vi "Write tSignalonTreeElements_Core.vi"(8 "error in (no error)":errorcluster, 9 "System_settings IN":T1={"Units in the system"=[], "dBase names by units"=[], "TCP/IP processing units addresses"=[], "TCP/IP server address"="", "dBase User Name_Cli"="codis_cli", "dBase User Password_Cli"="codis_cli", "dBase User Name_Med"="codis_med_wrt", "dBase User Password_Med"="codis_med_wrt", "Sampling rate [Hz]"=0.0, "FTP Server User name, cRIO"="", "FTP Server Password, cRIO"="", "OnScreenKeyboardPopUp"=FALSE, "Number of points to collect"=0, "Main Window has title bar?"=FALSE, "Demo?"=FALSE, "dBase - Limit # of  elements to read"=0, "dBase Backup"={"dBase Backup Base Folder"="c:\\codis\\backup\\", "Remote dBase Backup Configured?"=TRUE}, "System Status"={"System Monitor Refresh Rate (ms)"=10000, "System Status Log  File"="c:\\codis\\system_info.txt", "Max number of elements to read\n"=26611200}, "Number of points to average for stationary state"=[60], "Number of points to collect for saving waveforms per channel"=[60], "Sources per Unit"=[], "TCP/IP_client_mediator_communication ports"=2058, "TCP/IP processing_units _mediator_communication ports"=2055}, 10 "1D array of Pan Cluster IN":T4[](array[typedef]) {"Absolute Minimum Air Gap per Plane"."Absolute AG Minimum Pole Number" format="%.3f"; "Absolute Minimum Air Gap per Plane"."Absolute AG Minimum Value" format="%.3f"; "Magnetic Field Data"."Maximum by Pole Number" format="%.3f"; "Air Gap Data"."Minimum by Pole Number" format="%.3f"; "Orbit(s) - XY"."Orbit XY Graphs (Synthesized from Selected Harmonics and DC)"."?" format="%.3f"; "Orbit(s) - XY"."Orbit XY Graphs (Synthesized from Selected Harmonics and DC)"."?" format="%.3f"; "Orbit(s) - XY"."Orbit XY Graphs (Glided and Averaged on One Revolution)"."?" format="%.3f"; "Orbit(s) - XY"."Orbit XY Graphs (Glided and Averaged on One Revolution)"."?" format="%.3f"; "Orbit(s) - XY"."Orbit XY Graphs (Unaveraged)"."?" format="%.3f"; "Orbit(s) - XY"."Orbit XY Graphs (Unaveraged)"."?" format="%.3f"}) -> ()   [LabVIEW 2014]
uses:
  common/typedefs/Pan_Cluster_Core.ctl
  common/typedefs/Condition_Vector_Cluster_Core.ctl
  common/typedefs/Unit_Names_Core.ctl
  common/typedefs/Data_Sources_Core.ctl
  common/typedefs/System_Settings_Cluster_Client_Mediator_Core.ctl
  <vilib>/addons/database/Connection.llb/DB Tools Open Connec (String).vi
  <vilib>/addons/database/_DB Variant To Data/Database Variant To Data.xnode
  <vilib>/addons/database/NI_Database_API.lvlib
panel:
  out "SignalLabel OUT":string[](array[string])
  out "TreeCategoryName":string[](array[string])
  out "idtTreeCategories OUT":u32[](array[numeric])
  out "TreeCategoryLabel":string[](array[string])
  out "error out 2":errorcluster
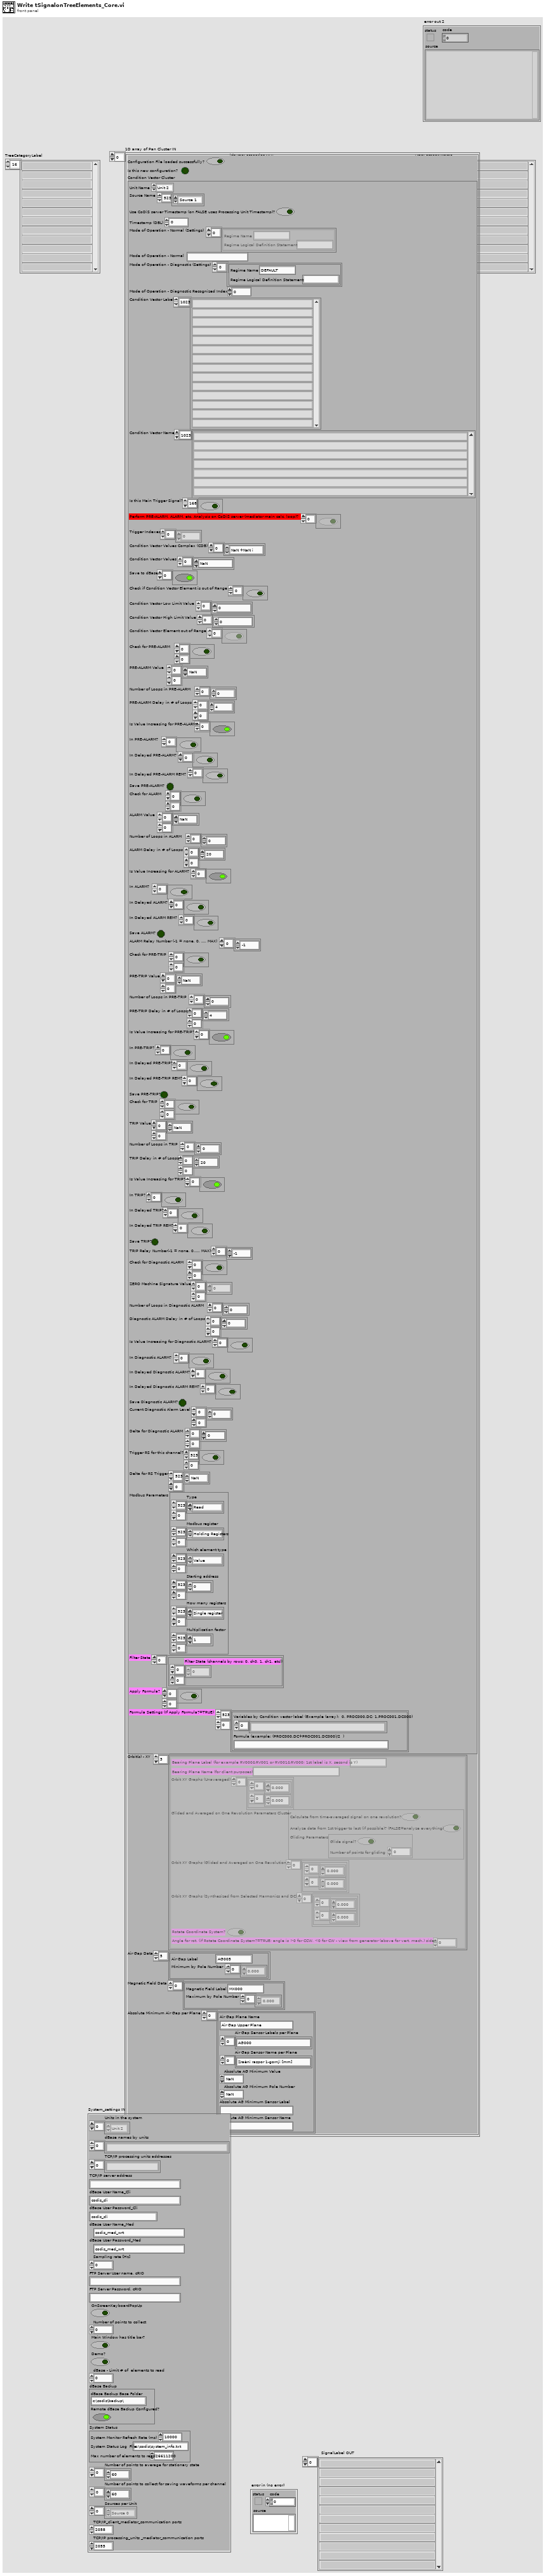
[diagram p1: front panel]
types:
  T1 = typedef "System_Settings_Cluster_Client_Mediator_Core.ctl" = cluster{"Units in the system":T2[], "dBase names by units":string[], "TCP/IP processing units addresses":string[], "TCP/IP server address":string, "dBase User Name_Cli":string, "dBase User Password_Cli":string, "dBase User Name_Med":string, "dBase User Password_Med":string, "Sampling rate [Hz]":dbl, "FTP Server User name, cRIO":string, "FTP Server Password, cRIO":string, "OnScreenKeyboardPopUp":bool, "Number of points to collect":u32, "Main Window has title bar?":bool, "Demo?":bool, "dBase - Limit # of  elements to read":u32, "dBase Backup":cluster{"dBase Backup Base Folder":string, "Remote dBase Backup Configured?":bool}, "System Status":cluster{"System Monitor Refresh Rate (ms)":u32, "System Status Log  File":string, "Max number of elements to read\n":i64}, "Number of points to average for stationary state":i32[], "Number of points to collect for saving waveforms per channel":i32[], "Sources per Unit":T3[], "TCP/IP_client_mediator_communication ports":u16, "TCP/IP processing_units _mediator_communication ports":u16}
  T2 = typedef "Unit_Names_Core.ctl" = enum16{"Not used", "Unit 1", "Unit 2", "Unit 3", "Unit 4", "Unit 5", "Unit 6", "Unit 7", "Unit 8", "Unit 9"}
  T3 = typedef "Data_Sources_Core.ctl" = enum16{"Not Used", "Source 0", "Source 1", "Source 2", "Source 3", "Source 4", "Source 5", "Source 6", "Source 7", "Source 8", "Source 9", "Source 10", "Source 11", "Source 12", "Source 13", "Source 14", "Source 15", "Source 16", "Source 17", "Source 18", "Source 19", "Source 20"}
  T4 = typedef "Pan_Cluster_Core.ctl" = cluster{"Configuration File loaded successfully?":bool, "Is this new configuration?":bool, "Condition Vector Cluster":T5, "Orbit(s) - XY":cluster{"Bearing Plane Label (for example RV000&RV001 or RV001&RV000; 1st label is X, second is Y)":string, "Bearing Plane Name (for client purposes)":string, "Orbit XY Graphs (Unaveraged)":cluster{sgl[], sgl[]}[], "Glided and Averaged on One Revolution Parameters Cluster":cluster{"Calculate from time-averaged signal on one revolution?":bool, "Analyze data from 1st trigger to last (if possible)? (FALSE=analyze everything)":bool, "Gliding Parameters":cluster{"Glide signal?":bool, "Number of points for gliding":u16}}, "Orbit XY Graphs (Glided and Averaged on One Revolution)":cluster{sgl[], sgl[]}[], "Orbit XY Graphs (Synthesized from Selected Harmonics and DC)":cluster{sgl[], sgl[]}[], "Rotate Coordinate System?":bool, "Angle for rot. (if Rotate Coordinate System?=TRUE; angle is >0 for CCW, <0 for CW - view from generator (above for vert. mach.) side)":sgl}[], "Air Gap Data":cluster{"Air Gap Label":string, "Minimum by Pole Number":sgl[]}[], "Magnetic Field Data":cluster{"Magnetic Field Label":string, "Maximum by Pole Number":sgl[]}[], "Absolute Minimum Air Gap per Plane":cluster{"Air Gap Plane Name":string, "Air Gap Sensor Labels per Plane":string[], "Air Gap Sensor Name per Plane":string[], "Absolute AG Minimum Value":sgl, "Absolute AG Minimum Pole Number":sgl, "Absolute AG Minimum Sensor Label":string, "Absolute AG Minimum Sensor Name":string}[]}
  T5 = typedef "Condition_Vector_Cluster_Core.ctl" = cluster{"Unit Name":T2, "Source Name":T3[], "Use CoDiS server Timestamp (on FALSE uses Processing Unit Timestamp)?":bool, "Timestamp (DBL)":dbl, "Mode of Operation - Normal (Settings)":cluster{"Regime Name":string, "Regime Logical Definition Statement":string}[], "Mode of Operation - Normal":string, "Mode of Operation - Diagnostic (Settings)":cluster{"Regime Name":string, "Regime Logical Definition Statement":string}[], "Mode of Operation - Diagnostic Recognized Index":i16, "Condition Vector Label":string[], "Condition Vector Name":string[], "Is this Main Trigger Signal?":bool[], "Perform PRE-ALARM, ALARM, etc. Analysis on CoDiS server (mediator main calc. loop)?":bool[], "Trigger Indexes":u32[], "Condition Vector Values Complex (CDB)":cdb[], "Condition Vector Values":sgl[], "Save to dBase":bool[], "Check if Condition Vector Element is out of Range":bool[], "Condition Vector Low Limit Value":sgl[], "Condition Vector High Limit Value":sgl[], "Condition Vector Element out of Range":bool[], "Check for PRE-ALARM":bool[][], "PRE-ALARM Value":sgl[][], "Number of Loops in PRE-ALARM":u32[], "PRE-ALARM Delay in # of Loops":u16[][], "Is Value Increasing for PRE-ALARM?":bool[], "In PRE-ALARM?":bool[], "In Delayed PRE-ALARM?":bool[], "In Delayed PRE-ALARM REM?":bool[], "Save PRE-ALARM?":bool, "Check for ALARM":bool[][], "ALARM Value":sgl[][], "Number of Loops in ALARM":u32[], "ALARM Delay in # of Loops":u16[][], "Is Value Increasing for ALARM?":bool[], "In ALARM?":bool[], "In Delayed ALARM?":bool[], "In Delayed ALARM REM?":bool[], "Save ALARM?":bool, "ALARM Relay Number (-1 = none, 0, ..., MAX)":i16[], "Check for PRE-TRIP":bool[][], "PRE-TRIP Value":sgl[][], "Number of Loops in PRE-TRIP":u32[], "PRE-TRIP Delay in # of Loops":u16[][], "Is Value Increasing for PRE-TRIP?":bool[], "In PRE-TRIP?":bool[], "In Delayed PRE-TRIP?":bool[], "In Delayed PRE-TRIP REM?":bool[], "Save PRE-TRIP?":bool, "Check for TRIP":bool[][], "TRIP Value":sgl[][], "Number of Loops in TRIP":u32[], "TRIP Delay in # of Loops":u16[][], "Is Value Increasing for TRIP?":bool[], "In TRIP?":bool[], "In Delayed TRIP?":bool[], "In Delayed TRIP REM?":bool[], "Save TRIP?":bool, "TRIP Relay Number(-1 = none, 0,..., MAX)":i16[], "Check for Diagnostic ALARM":bool[][], "ZERO Machine Signature Value":dbl[][], "Number of Loops in Diagnostic ALARM":u32[], "Diagnostic ALARM Delay in # of Loops":u16[][], "Is Value Increasing for Diagnostic ALARM?":bool[], "In Diagnostic ALARM?":bool[], "In Delayed Diagnostic ALARM?":bool[], "In Delayed Diagnostic ALARM REM?":bool[], "Save Diagnostic ALARM?":bool, "Current Diagnostic Alarm Level":sgl[][], "Delta for Diagnostic ALARM":sgl[][], "Trigger RS for this channel?":bool[][], "Delta for RS Trigger":sgl[][], "Modbus Parameters":cluster{"Type":enum16{"Read", "Write", "None"}[][], "Modbus register":enum16{"Coils", "Discrete Inputs", "Input Registers", "Holding Registers"}[][], "Which element type":enum16{"Value", "Alarm", "Trip"}[][], "Starting address":u16[][], "How many registers":enum16{"Single register", "HI-LO", "LO-HI"}[][], "Multiplication factor":dbl[][]}, "Filter State":cluster{"Filter State (channels by rows: 0. ch0, 1. ch1, etc))":dbl[][]}[], "Apply Formula?":bool[][], "Formula Settings (If Apply Formula?=TRUE)":cluster{"Variables by Condition vector label (Example (array):  0. PROC000.DC; 1.PROC001.DC000)":string[], "Formula (example: (PROC000.DC+PROC001.DC000)/2  )":string}[][]}
  T6 = typedef "NI_Database_API.lvlib/Conn ObjectReference.ctl" = refnum<k1>
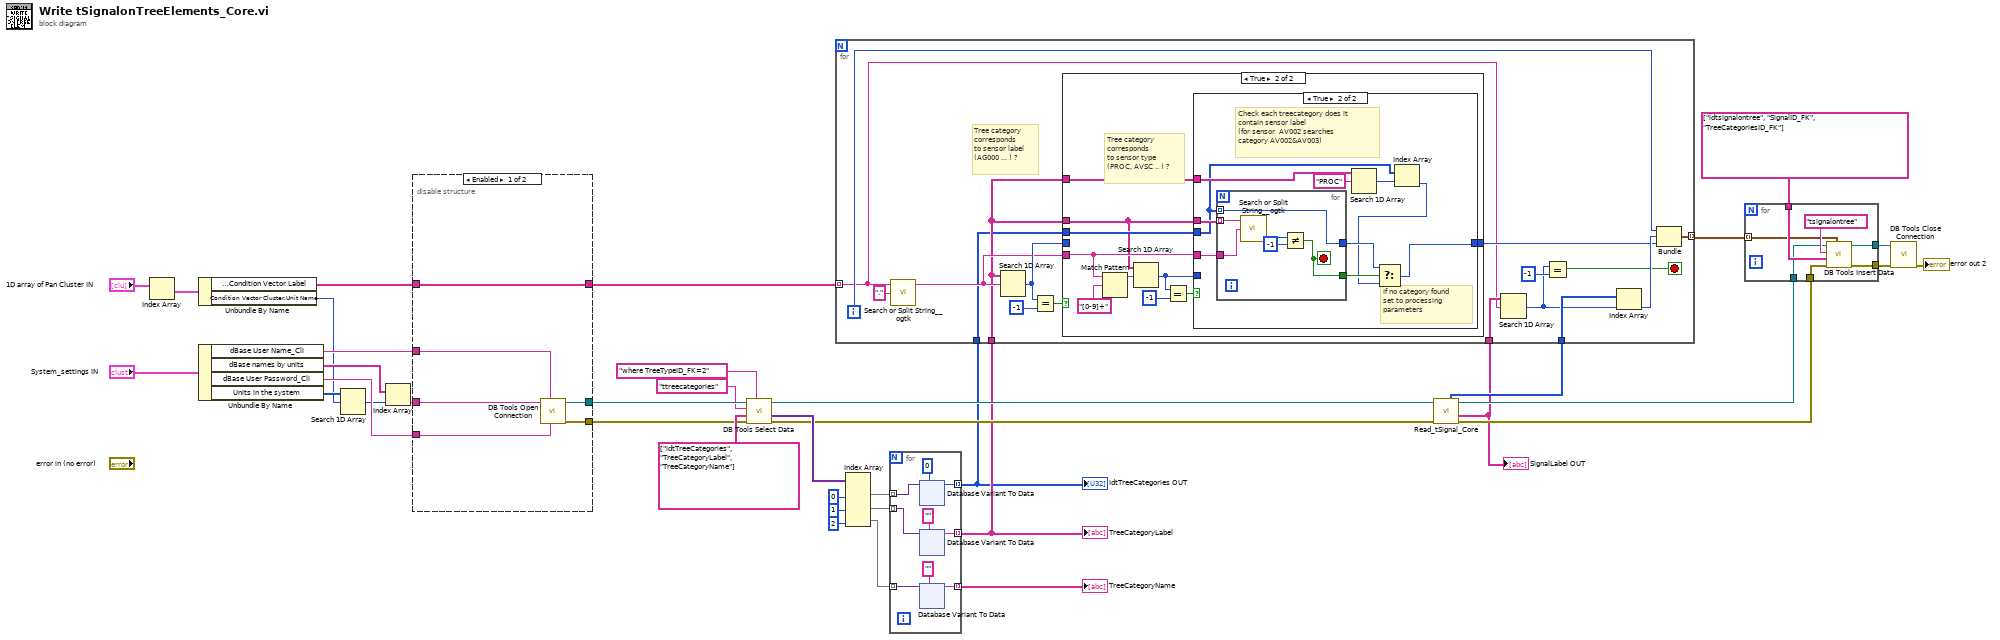
[diagram p0: block diagram]
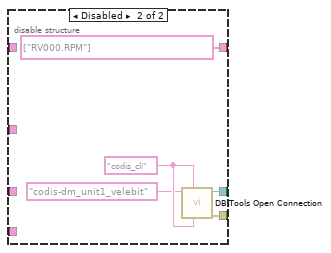
[diagram p2: hidden frame]
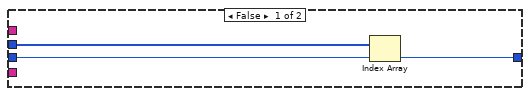
[diagram p3: hidden frame]
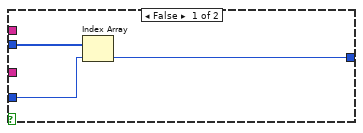
[diagram p4: hidden frame]
diagram:
  n1 = Index Array(array="1D array of Pan Cluster IN") -> (element=w38:T4)  [unwired: 1 in]
  n2 = Unbundle By Name(w38) -> ("Condition Vector Cluster.Condition Vector Label"=w2:string[], "Condition Vector Cluster.Unit Name"=w29:T2)
  n3 = Unbundle By Name("System_settings IN") -> ("dBase User Name_Cli"=w35:string, "dBase names by units"=w36:string[], "dBase User Password_Cli"=w34:string, "Units in the system"=w33:T2[])
  n4 = Search 1D Array(1D array=w33, element=w29) -> (index of element=w32:i32)  [unwired: 1 in]
  n5 = Index Array(array=w36, index=w32) -> (element=w37:string)
  n6 = disable-structure shown="Enabled" {
    disable-tunnel: w37 -> [w44 _]
    disable-tunnel: w35 -> [w43 _]
    disable-tunnel: w34 -> [w42 _]
    disable-tunnel: [w41 w49] -> w17
    disable-tunnel: [w40 w48] -> w16
    disable-tunnel: [w39 string[] ["RV000.RPM"] ("Condition Vector Label")] -> w3
    disable-tunnel: w2 -> [w39 _]
    frame Enabled {
      n7 = call-poly <vilib>:"DB Tools Open Connection.vi"("password"=w42, "userID"=w43, "connection information"=w44) -> ("error out"=w40:errorcluster, "connection reference"=w41:T6)  [unwired: 5 in]
    }
    frame Disabled {
      w47 = "codis_cli" ("dBase User Password_Cli")
      n8 = call-poly <vilib>:"DB Tools Open Connection.vi"("password"=w47, "userID"=w47, "connection information"="codis-dm_unit1_velebit" ("dBase Name")) -> ("error out"=w48:errorcluster, "connection reference"=w49:T6)  [unwired: 5 in]
    }
  }
  n9 = call <vilib>:"DB Tools Select Data.vi"("condition"="where TreeTypeID_FK=2", "error in (no error)"=w16, "columns"=string[] ["idtTreeCategories", "TreeCategoryLabel", "TreeCategoryName"], "table"="ttreecategories", "connection reference"=w17) -> ("error out"=w12:errorcluster, "data"=w24:variant[][], "connection reference out"=w13:T6)  [unwired: 1 in]
  n10 = Index Array(array=w24, index (col) #1=0 ("disabled index (col)"), index (col) #2=1 ("index (col)"), index (col) #3=2 ("index (col)")) -> (element #1=w26:variant[], element #2=w22:variant[], element #3=w19:variant[])  [unwired: 3 in]
  n11 = for {
    tunnel: w26 -> [w58] mode=indexing
    tunnel: [w57] -> w10 mode=indexing
    tunnel: [w54] -> w11 mode=indexing
    tunnel: w22 -> [w53] mode=indexing
    tunnel: w19 -> [w51] mode=indexing
    tunnel: [w50] -> w18 mode=indexing
    n12 = xnode "Database Variant To Data"("database variant"=w58, "type"=u32 0) -> ("data"=w57:u32)  [unwired: 1 in, 1 out]
    n13 = xnode "Database Variant To Data"("database variant"=w53, "type"="") -> ("data"=w54:string)  [unwired: 1 in, 1 out]
    n14 = xnode "Database Variant To Data"("database variant"=w51, "type"="") -> ("data"=w50:string)  [unwired: 1 in, 1 out]
  }
  "TreeCategoryLabel" <- w11
  "idtTreeCategories OUT" <- w10
  "TreeCategoryName" <- w18
  n15 = call "Read_tSignal_Core.vi"("error in (no error)"=w12, "connection reference IN"=w13) -> ("error out"=w27:errorcluster, "SignalLabel OUT"=w1:string[], "connection reference OUT"=w28:T6, "idtSignal OUT"=w31:u16[])  [unwired: 5 in, 1 out]
  "SignalLabel OUT" <- w1
  n16 = for {
    tunnel: w3 -> [w164] mode=indexing
    tunnel: w11 -> [w156]
    tunnel: w10 -> [w155]
    tunnel: w1 -> [w171]
    tunnel: w31 -> [w169]
    tunnel: [w166] -> w30 mode=indexing
    i -> [w170]
    stop <- w158 stop-if-true
    # "Tree category \ncorresponds\nto sensor label\n(AG000 ... ) ?"
    n17 = call <userlib>:"Search or Split String__ogtk.vi"("search string/char (-)"=".", "string"=w164) -> ("substring before match"=w157:string)  [unwired: 1 in, 2 out]
    n18 = Search 1D Array(1D array=w156, element=w157) -> (index of element=w163:i32)  [unwired: 1 in]
    n19 = Equal?(x=w163, y=-1) -> (x = y?=w161:bool)
    n20 = case shown="True" w161 {
      tunnel: w155 -> [w174 w184]
      tunnel: [w173 w183] -> w167
      tunnel: w163 -> [w172 _]
      tunnel: w156 -> [_ w180]
      tunnel: w157 -> [_ w181]
      tunnel: w156 -> [_ w175]
      frame False {
        n21 = Index Array(array=w174, index=w172) -> (element=w173:u32)
      }
      frame True {
        # "Tree category \ncorresponds\nto sensor type\n(PROC, AVSC .. ) ?"
        n22 = Match Pattern(string=w181, regular expression="[0-9]+") -> (before substring=w179:string)  [unwired: 1 in, 3 out]
        n23 = Search 1D Array(1D array=w180, element=w179) -> (index of element=w176:i32)  [unwired: 1 in]
        n24 = Equal?(x=w176, y=-1) -> (x = y?=w177:bool)
        n25 = case shown="True" w177 {
          tunnel: w184 -> [w187 w190]
          tunnel: [w185 w188] -> w183
          tunnel: w181 -> [_ w197]
          tunnel: w180 -> [_ w196]
          tunnel: w176 -> [w186 _]
          tunnel: w175 -> [_ w195]
          frame False {
            n26 = Index Array(array=w187, index=w186) -> (element=w185:u32)
          }
          frame True {
            # "If no category found\nset to processing\nparameters"
            # "Check each treecategory does it \ncontain sensor label\n(for sensor  AV002 searches\ncategory AV002&AV003)"
            n27 = for {
              tunnel: w196 -> [w203] mode=indexing
              tunnel: w197 -> [w202]
              tunnel: w190 -> [w199] mode=indexing
              tunnel: [w199] -> w192
              tunnel: [w198] -> w193
              stop <- w198 stop-if-true
              n28 = call <userlib>:"Search or Split String__ogtk.vi"("search string/char (-)"=w202, "string"=w203) -> ("offset after match"=w201:i32)  [unwired: 1 in, 2 out]
              n29 = Not Equal?(x=w201, y=-1) -> (x != y?=w198:bool)
            }
            n30 = Search 1D Array(1D array=w195, element="PROC") -> (index of element=w191:i32)  [unwired: 1 in]
            n31 = Index Array(array=w190, index=w191) -> (element=w189:u32)
            n32 = Select(t=w192, s=w193, f=w189) -> (s? t:f=w188:u32)
          }
        }
      }
    }
    n33 = Search 1D Array(1D array=w171, element=w164) -> (index of element=w159:i32)  [unwired: 1 in]
    n34 = Equal?(x=w159, y=-1) -> (x = y?=w158:bool)
    n35 = Index Array(array=w169, index=w159) -> (element=w168:u16)
    n36 = Bundle(w170, "data"=w168, "data"=w167) -> (w166:cluster{i32, "data":u16, "data":u32})  [unwired: 1 in]
  }
  n37 = for {
    tunnel: string[] ["idtsignalontree", "SignalID_FK", "TreeCategoriesID_FK"] ("columns") -> [w209]
    tunnel: w28 -> [w208]
    tunnel: w27 -> [w207]
    tunnel: [w206] -> w5
    tunnel: w30 -> [w205] mode=indexing
    tunnel: [w204] -> w6
    n38 = call <vilib>:"DB Tools Insert Data.vi"("data"=w205, "error in (no error)"=w207, "columns"=w209, "table"="tsignalontree", "connection reference"=w208) -> ("error out"=w206:errorcluster, "connection reference out"=w204:T6)  [unwired: 5 in]
  }
  n39 = call <vilib>:"DB Tools Close Connection.vi"("error in (no error)"=w5, "connection reference"=w6) -> ("error out"=→"error out 2":errorcluster)  [unwired: 5 in]
